vi "Rotate Drive.vi"() -> ()   [LabVIEW 2016]
uses:
  Refname/Sensors.ctl
  Refname/Refname to String (Sensors).vi
panel:
  out "error out":errorcluster
  in  "error in":errorcluster
  in  "Rotational Input":dbl format="%#_13g"
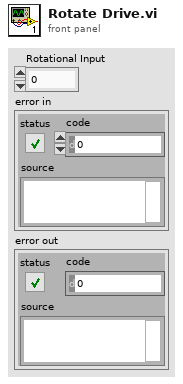
[diagram p1: front panel]
types:
  T1 = typedef "Sensors.ctl" = enum16{"DIP 1", "DIP 2", "DIP 3", "DIP 4", "Gyro"}
  T2 = typedef "WPI_GyroDevRef.ctl" = cluster{"DevStatus":errorcluster, "Analog Channel":T3, "Offset":dbl, "Gain (VoltsPerDegree/Second)":dbl, "Gyro Type":enum16{"Analog", "XRS450"}, "Handle":i32, "SPI Bus":T4, "Device Found":bool, "Sample Rate":dbl, "Calibrate On Open":bool}
  T3 = typedef "FPGA_AIChannel.ctl" = enum8{"AI 0", "AI 1", "AI 2", "AI 3", "AI MXP 0", "AI MXP 1", "AI MXP 2", "AI MXP 3", "Invalid"}
  T4 = typedef "spi_bus.ctl" = enum16{"SPI On-Board, CS0", "SPI On-Board, CS1", "SPI On-Board, CS2", "SPI On-Board, CS3", "SPI MXP", "Invalid"}
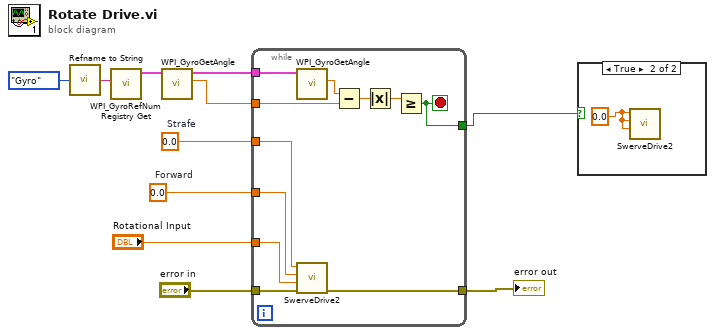
[diagram p0: block diagram]
diagram:
  w5 = 0.0  # Forward
  w4 = 0.0  # Strafe
  n1 = call-poly "Refname to String.vi"("Enum"=Sensors."Gyro") -> ("String"=w10:string)
  n2 = call <vilib>:"WPI_GyroRefNum Registry Get.vi"("refnum name"=w10) -> ("GyroDevRef"=w9:T2)  [unwired: 9 in, 1 out]
  n3 = call <vilib>:"WPI_GyroGetAngle.vi"("GyroDevRef"=w9) -> ("Angle"=w8:dbl, "GyroDevRef"=w7:T2)  [unwired: 6 in, 3 out]
  n4 = while {
    tunnel: w8 -> [w19]
    tunnel: w7 -> [w22]
    tunnel: "Rotational Input" -> [w17]
    tunnel: w5 -> [w16]
    tunnel: w4 -> [w15]
    tunnel: "error in" -> [w14]
    tunnel: [w13] -> w2
    tunnel: [w12] -> w1
    stop <- w12 stop-if-true
    n5 = call <vilib>:"WPI_GyroGetAngle.vi"("GyroDevRef"=w22) -> ("Angle"=w18:dbl)  [unwired: 6 in, 4 out]
    n6 = call "SwerveDrive2.vi"("error in"=w14, "Rotate"=w17, "Forward"=w16, "Strafe"=w15) -> ("error out"=w13:errorcluster)  [unwired: 7 in]
    n7 = Subtract(x=w18, y=w19) -> (x-y=w21:dbl)
    n8 = Absolute Value(x=w21) -> (abs(x)=w20:dbl)
    n9 = Greater Or Equal?(x=w20) -> (x >= y?=w12:bool)  [unwired: 1 in]
  }
  "error out" <- w2
  n10 = case shown="True" w1 {
    frame False {
    }
    frame True {
      w23 = 0.0 ("Rotate")
      n11 = call "SwerveDrive2.vi"("Rotate"=w23, "Forward"=w23, "Strafe"=w23) -> ()  [unwired: 8 in, 1 out]
    }
  }
